vi "Spray_tempcontrol_off.vi"(8 "error in (no error)":errorcluster) -> (0 "error out":errorcluster)   [LabVIEW 2015]
uses:
  <vilib>/httpClient/LabVIEWHTTPClient.lvlib
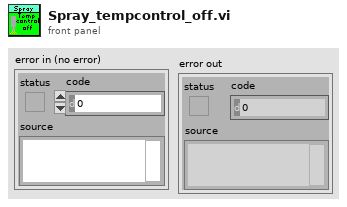
[diagram p1: front panel]
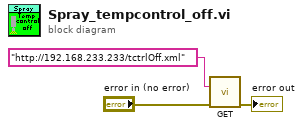
[diagram p0: block diagram]
diagram:
  n1 = call <vilib>:"GET.vi"("url"="http://192.168.233.233/tctrlOff.xml", "error in (no error)"="error in (no error)") -> ("error out"=→"error out":errorcluster)  [unwired: 10 in, 3 out]
